vi "MGCC_FntStaMach_system_time.vi"   [LabVIEW 2016]
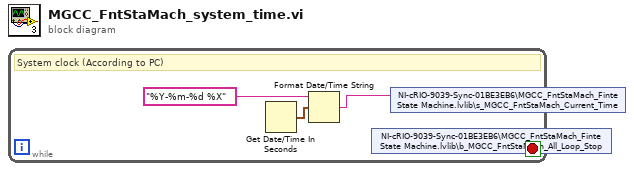
[diagram p0: block diagram]
diagram:
  n1 = while {
    stop <- w2 stop-if-true
    # "System clock (According to PC)"
    n2 = Get Date/Time In Seconds() -> (seconds since 1Jan1904=w4:timestamp)
    n3 = Format Date/Time String(time format string (%c)="%Y-%m-%d %X", seconds (now)=w4) -> (date/time string=w1:string)  [unwired: 1 in]
    n4 = shared-variable "NI-cRIO-9039-Sync-01BE3EB6\\MGCC_FntStaMach_Finte State Machine.lvlib\\b_MGCC_FntStaMach_All_Loop_Stop"() -> (w2:bool)  [unwired: 1 in, 1 out]
    n5 = shared-variable "NI-cRIO-9039-Sync-01BE3EB6\\MGCC_FntStaMach_Finte State Machine.lvlib\\s_MGCC_FntStaMach_Current_Time"(w1) -> ()  [unwired: 1 in, 1 out]
  }
